vi "Read Multi-Point [MP].vi"(8 "error in (no error)":errorcluster, 9 "array size":i32, 10 "maximum time (5s)":dbl[unit]=5000.0 caption="maximum time (5000 ms)", 11 "IVI_DMM in":refnum<class "IVI_DMM.lvclass">) -> (0 "error out":errorcluster, 1 "actual number of points":i32, 2 "reading array":dbl[](array[numeric]) format="%^.2e", 3 "IVI_DMM out":refnum<class "IVI_DMM.lvclass">)   [LabVIEW 2013, in "IVI_DMM.lvlib" / "IVI_DMM.lvclass"]
doc: "This VI initiates the measurement, waits for the DMM to return to the Idle state, and returns an array of measured values. The number of measurements the DMM takes is determined by the values you specify for the Trigger Count and Sample Count parameters of the IviDmm Configure Multi-Point [MP] VI.\n\nThis VI applies default values to properties that have not been set by the user under the following conditions:\n\n(1) If the user has not set the value of any property in the IviDmmMultiPoint extension group, the VI sets the IviDmm>>Multi-Point Acquisition>>Sample Count [MP] and IviDmm>>Multi-Point Acquisition>>Trigger Count [MP] properties to 1.\n\n(2) If the user has not set the value of the IviDmm>Measurement Operation Options>Auto Zero [AZ] property, the VI sets the value of this property to IVIDMM_VAL_AUTO_ZERO_OFF (0). \n\nNotes:\n\n(1) This VI is part of the IviDmmMultiPoint [MP] extension group.\n\n(2) After this VI executes, each element in the Reading Array parameter is an actual reading or a value indicating that an over-range condition occurred.\n\n(3) If an over-range condition occurs, the corresponding Reading Array element contains an IEEE defined NaN (Not a Number) value and the VI returns the IVIDMM_WARN_OVER_RANGE (0x3FFA2001) warning code. \n\n(4) You can test each element in the Reading Array parameter for an over-range condition by calling the IviDmm Is Over-Range VI.\n\n(5) This VI performs interchangeability checking when the IviDmm>>Inherent IVI Settings>>User Options>>Interchange Check property is set to TRUE. If the IviDmm>>Inherent IVI Settings>>User Options>>Spy property is set to TRUE, you use the NI Spy utility to view interchangeability warnings. You use the IviDmm Get Next Interchange Warning VI to retrieve interchangeability warnings when the IviDmm>>Inherent IVI Settings>>User Options>>Spy property is set to FALSE. For more information about interchangeability checking, refer to the help text for the IviDmm>>Inherent IVI Settings>>User Options>>Interchange Check property.\n\n(6) The class driver initiates an array of simulated measurements when this VI is called and the IviDmm>>Inherent IVI Settings>>User Options>>Simulate property is set to TRUE and the IviDmm>>Inherent IVI Settings>>User Options>>Use Specific Simulation property is set to FALSE. For information on how to configure a simulated measurement, refer to the online help manual."
uses:
  IVI_DMM.lvclass
  IVI_DMM.lvclass/IVI_DMM.ctl
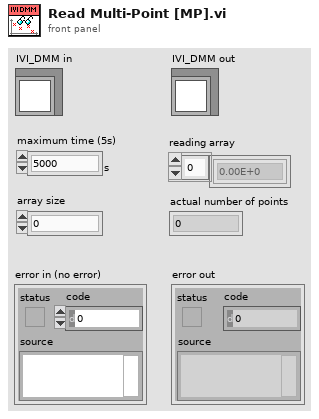
[diagram p1: front panel]
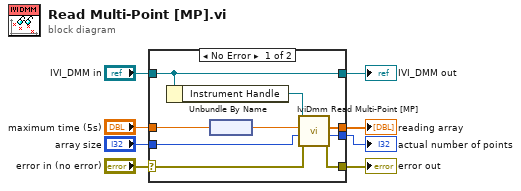
[diagram p0: block diagram]
diagram:
  n1 = case shown="No Error" "error in (no error)" {
    selector: "error in (no error)" -> [w15 w19]
    tunnel: [w14 w19] -> w7
    tunnel: [w17 w18] -> w5
    tunnel: "IVI_DMM in" -> [w17 w18]
    tunnel: "maximum time (5s)" -> [w13 _]
    tunnel: "array size" -> [w11 _]
    tunnel: [w10 _] -> w2
    tunnel: [w9 _] -> w1
    frame No Error {
      n2 = Unbundle By Name(w17) -> ("Instrument Handle"=w16:refnum<k15>)
      n3 = node(w13) -> (w12:dbl)
      n4 = call <vilib>:"IviDmm Read Multi-Point [MP].vi"("error in (no error)"=w15, "array size"=w11, "maximum time (5000 ms)"=w12, "instrument handle"=w16) -> ("error out"=w14:errorcluster, "actual number of points"=w9:i32, "reading array"=w10:dbl[])  [unwired: 4 in, 1 out]
    }
    frame Error {
    }
  }
  "error out" <- w7
  "IVI_DMM out" <- w5
  "reading array" <- w2
  "actual number of points" <- w1
